vi "Template - UEvent.vi"(7 "Event Selector":T2=enum."Generate U Event", 8 "error in (no error)":errorcluster, 10 "User Event Data":cluster{"Data Type":T1, "Data":variant}) -> (0 "error out":errorcluster, 2 "Event Reg Refnum":refnum<event-registration>, 3 "U-Event Refnum":T3)   [LabVIEW 2012]
uses:
  TypeDef - Template - UEvent Ref.ctl
  TypeDef - Template - UEvent Data Enum.ctl
  Navistar Library/Controls/TypeDef - UEvent Selector(Standard).ctl
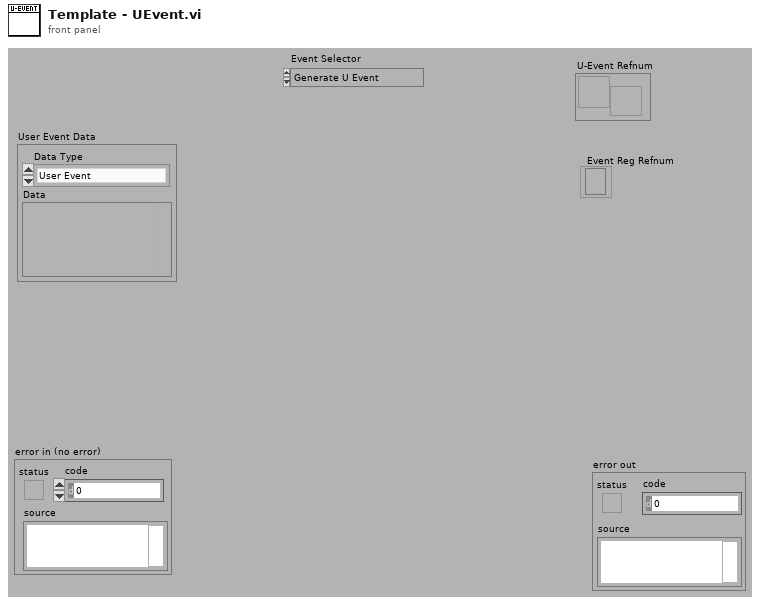
[diagram p1: front panel]
types:
  T1 = typedef "TypeDef - Template - UEvent Data Enum.ctl" = enum16{"User Event", "Stop"}
  T2 = typedef "TypeDef - UEvent Selector(Standard).ctl" = enum16{"Create UEvent", "Get UEvent Ref", "Clear UEvent", "Reset UEvent", "Generate U Event"}
  T3 = typedef "TypeDef - Template - UEvent Ref.ctl" = refnum<user-event>
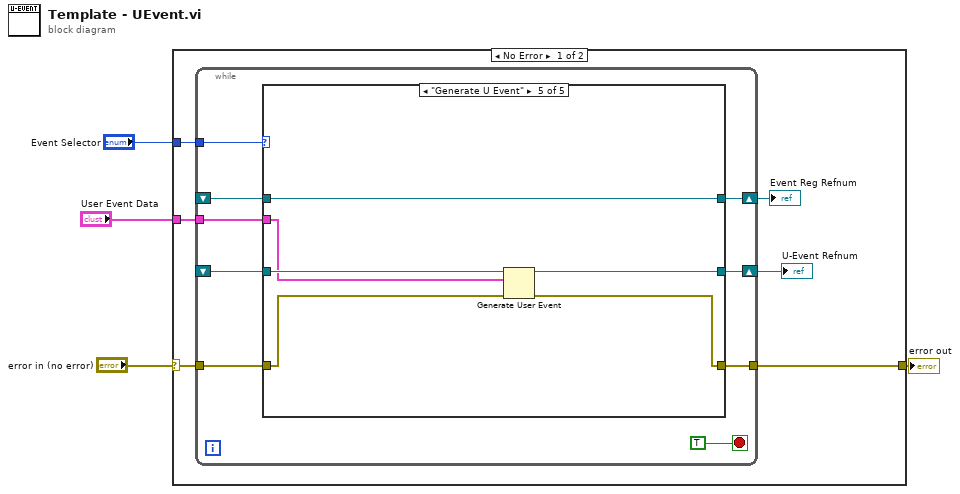
[diagram p0: block diagram]
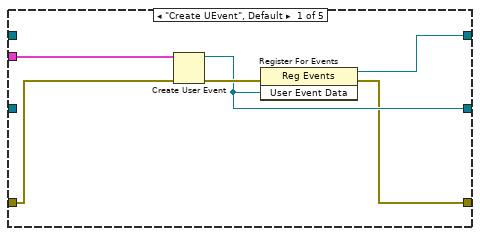
[diagram p2: hidden frame]
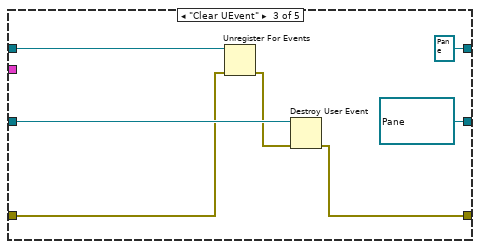
[diagram p4: hidden frame]
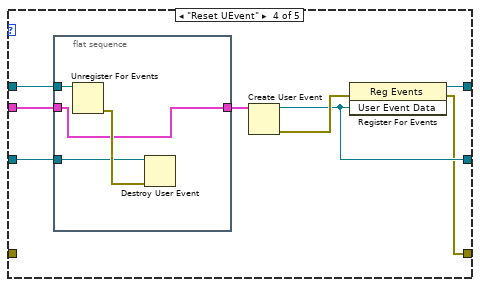
[diagram p5: hidden frame]
diagram:
  n1 = case shown="No Error" "error in (no error)" {
    selector: "error in (no error)" -> [w8 w54]
    tunnel: [w7 w54] -> w3
    tunnel: "Event Selector" -> [w6 _]
    tunnel: "User Event Data" -> [w5 _]
    frame No Error {
      n2 = while {
        shift-right: [w19] -> w9
        shift-left: _ -> [w15]
        shift-right: [w18] -> w10
        shift-left: _ -> [w14]
        tunnel: w8 -> [w17]
        tunnel: [w16] -> w7
        tunnel: w5 -> [w11]
        tunnel: w6 -> [w13]
        stop <- TRUE stop-if-true
        n3 = case shown="\"Generate U Event\"" w13 {
          tunnel: [w24 w28 refnum<event-registration> refnum ("Event Registration Refnum") w39 w49] -> w19
          tunnel: [w23 w27 refnum<user-event> refnum ("User Event Data") w38 w52] -> w18
          tunnel: w17 -> [w22 w26 w33 _ w51]
          tunnel: [w21 w26 w31 w37 w50] -> w16
          tunnel: w15 -> [_ w28 w34 w43 w49]
          tunnel: w14 -> [_ w27 w35 w42 w53]
          tunnel: w11 -> [w20 _ _ w36 w48]
          frame "Create UEvent", Default {
            n4 = Create User Event(user event datatype=w20, error in=w22) -> (user event=w23:refnum<user-event>, error out=w25:errorcluster)
            n5 = register-events(error in=w25, w23) -> (reference out=w24:refnum<event-registration>, error out=w21:errorcluster)  [unwired: 1 in]
          }
          frame "Get UEvent Ref" {
          }
          frame "Clear UEvent" {
            n6 = Unregister For Events(event registration refnum=w34, error in=w33) -> (error out=w32:errorcluster)
            n7 = Destroy User Event(user event=w35, error in=w32) -> (error out=w31:errorcluster)
          }
          frame "Reset UEvent" {
            n8 = flat-sequence {
              tunnel: w43 -> [w46]
              tunnel: w42 -> [w45]
              tunnel: [w44] -> w41
              tunnel: w36 -> [w44]
              frame #0 {
                n9 = Unregister For Events(event registration refnum=w46) -> (error out=w47:errorcluster)  [unwired: 1 in]
                n10 = Destroy User Event(user event=w45, error in=w47) -> ()  [unwired: 1 out]
              }
            }
            n11 = Create User Event(user event datatype=w41) -> (user event=w38:refnum<user-event>, error out=w40:errorcluster)  [unwired: 1 in]
            n12 = register-events(error in=w40, w38) -> (reference out=w39:refnum<event-registration>, error out=w37:errorcluster)  [unwired: 1 in]
          }
          frame "Generate U Event" {
            n13 = Generate User Event(user event=w53, event data cluster=w48, error in=w51) -> (user event out=w52:refnum<user-event>, error out=w50:errorcluster)
          }
        }
      }
      "U-Event Refnum" <- w10
      "Event Reg Refnum" <- w9
    }
    frame Error {
    }
  }
  "error out" <- w3
